vi "Get RemIO Read Scaling Factor.vi"(8 "error in (no error)":errorcluster, 10 "11102 in":refnum<class "11102.lvclass">, 11 "Node Ptr In":T1 format="%.0x") -> (0 "error out":errorcluster, 1 "Scaling Factors":dbl[](array[numeric]), 2 "11102 out":refnum<class "11102.lvclass">, 3 "Node Ptr Out":T1 format="%.0x", 5 "Per Channel?":bool)   [LabVIEW 2017, in "Modules.lvlib" / "11102.lvclass"]
doc: "This VI Returns the scaling factors for REM IO Input Modules"
uses:
  11102.lvclass
  <vilib>/NI Veristand/Custom Device API/Custom Device Item Ref.ctl
  11102.lvclass/11102.ctl
  <vilib>/indcomecat/Remote IO/internal/_Scale REM-11102.vi
  <vilib>/indcomecat/Remote IO/NI ECAT Remote IO.lvlib
  <vilib>/NI Veristand/Custom Device API/Custom Device API.lvlib
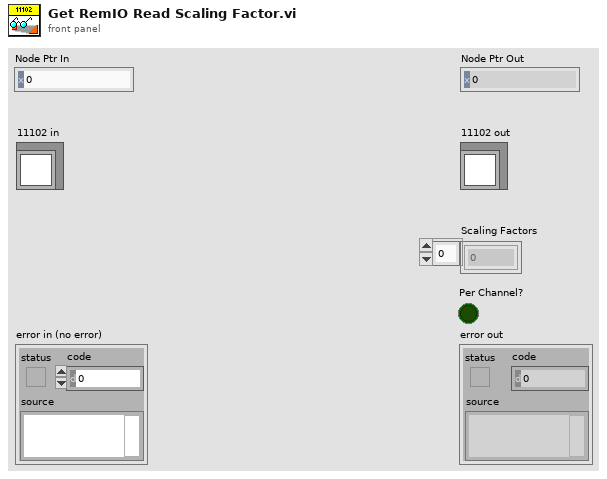
[diagram p1: front panel]
types:
  T1 = typedef "Custom Device API.lvlib/Custom Device Item Ref.ctl" = u64
  T2 = typedef "NI ECAT Remote IO.lvlib/channul number REM-11102.ctl" = u8
  T3 = typedef "NI ECAT Remote IO.lvlib/input filter time REM-11102.ctl" = u8
  T4 = typedef "NI ECAT Remote IO.lvlib/mean-value REM-11102.ctl" = u8
  T5 = typedef "NI ECAT Remote IO.lvlib/measuring range REM-11102.ctl" = u8
  T6 = cluster{"channel number":T2, "input filter time":T3, "mean-value":T4, "measuring range":T5}[]
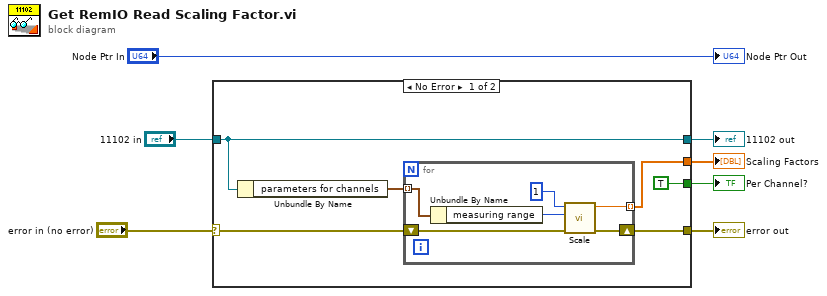
[diagram p0: block diagram]
diagram:
  n1 = case shown="No Error" "error in (no error)" {
    selector: "error in (no error)" -> [w13 w21]
    tunnel: [w11 w21] -> w6
    tunnel: [w9 w20] -> w3
    tunnel: "11102 in" -> [w9 w20]
    tunnel: [w10 _] -> w1
    tunnel: [TRUE _] -> w2
    frame No Error {
      n2 = Unbundle By Name(w9) -> ("parameters for channels"=w8:T6)
      n3 = for {
        shift-right: [w18] -> w11
        shift-left: w13 -> [w19]
        tunnel: [w17] -> w10 mode=indexing
        tunnel: w8 -> [w16] mode=indexing
        n4 = Unbundle By Name(w16) -> ("measuring range"=w15:T5)
        n5 = call-poly <vilib>:"Scale.vi"("error in (no error)"=w19, "measuring range"=w15, "raw data"=u16 1) -> ("error out"=w18:errorcluster, "scaled data"=w17:dbl)  [unwired: 7 in]
      }
    }
    frame Error {
    }
  }
  "error out" <- w6
  "11102 out" <- w3
  "Scaling Factors" <- w1
  "Per Channel?" <- w2
  "Node Ptr Out" <- "Node Ptr In"
